vi "GetDataPackage_Binary.vi"(8 "error in (no error)":errorcluster, 11 "VISA Refnum in":refnum<visa-resource-name>) -> (0 "error out":errorcluster, 1 "Raw Data":string, 2 "Data":T1[](array[typedef]), 3 "VISA Refnum out":refnum<visa-resource-name>)   [LabVIEW 2020, in "OXYGEN_Datastream.lvlib"]
uses:
  OXYGEN_Datastream.lvlib
  TypeDefs/DataPoint_Binary.ctl
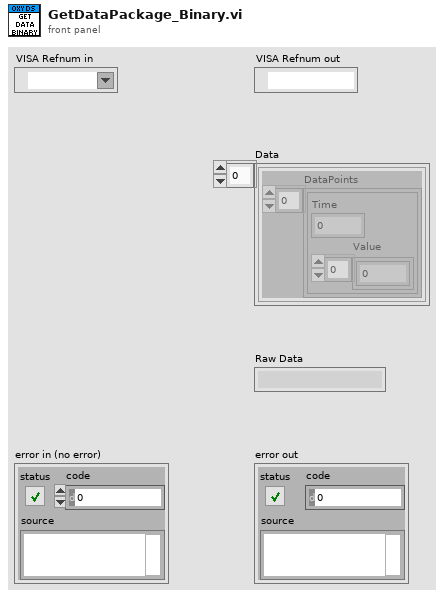
[diagram p1: front panel]
types:
  T1 = typedef "OXYGEN_Datastream.lvlib/DataPoint_Binary.ctl" = cluster{"DataPoints":cluster{"Time":dbl, "Value":u8[]}[]}
  T2 = typedef "OXYGEN_Datastream.lvlib/DataPoint_Variant.ctl" = cluster{"DataPoints":cluster{"Time":dbl, "Value":variant}[]}
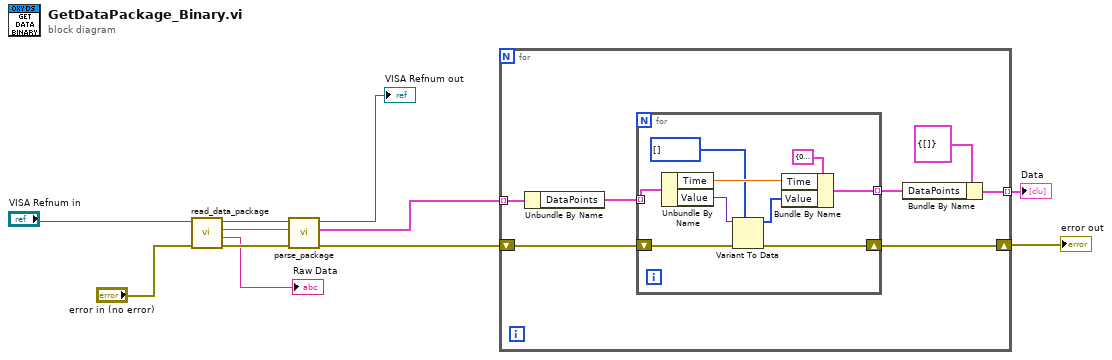
[diagram p0: block diagram]
diagram:
  n1 = call "read_data_package.vi"("error in (no error)"="error in (no error)", "OXY_SCPI Reseource In"="VISA Refnum in") -> ("error out"=w6:errorcluster, "Complete Raw data"=→"Raw Data":string, "Package without Header"=w8:string, "OXY_SCPI Reseource Out"=w7:refnum<visa-resource-name>)  [unwired: 6 in]
  n2 = call "parse_package.vi"("error in (no error)"=w6, "Raw Package without Header"=w8, "OXY_SCPI Reseource In"=w7) -> ("error out"=w4:errorcluster, "DataAllChannels"=w5:T2[], "OXY_SCPI Reseource Out"=→"VISA Refnum out":refnum<visa-resource-name>)  [unwired: 6 in]
  n3 = for {
    tunnel: w5 -> [w18] mode=indexing
    shift-right: [w15] -> w3
    shift-left: w4 -> [w16]
    tunnel: [w13] -> w2 mode=indexing
    n4 = Unbundle By Name(w18) -> ("DataPoints"=w17:cluster{"Time":dbl, "Value":variant}[])
    n5 = for {
      tunnel: w17 -> [w27] mode=indexing
      shift-right: [w24] -> w15
      shift-left: w16 -> [w25]
      tunnel: [w23] -> w14 mode=indexing
      n6 = Unbundle By Name(w27) -> ("Time"=w26:dbl, "Value"=w22:variant)
      n7 = Variant To Data(error in=w25, type=u8[] [], Variant=w22) -> (data=w20:u8[], error out=w24:errorcluster)
      n8 = Bundle By Name(cluster=cluster{"Time":dbl, "Value":u8[]} {"Time"=0.0, "Value"=[]}, "Time"=w26, "Value"=w20) -> (w23:cluster{"Time":dbl, "Value":u8[]})
    }
    n9 = Bundle By Name(cluster=T1 {"DataPoints"=[]} ("Data"), "DataPoints"=w14) -> (w13:T1)
  }
  "error out" <- w3
  "Data" <- w2
